vi "ktc11.vi"() -> ()   [LabVIEW 2018]
panel:
  out "RAW":dbl
  in  "stop":bool
  out "TANK":dbl(slide) scale=0.0..25.0
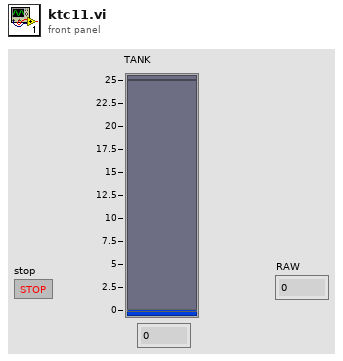
[diagram p1: front panel]
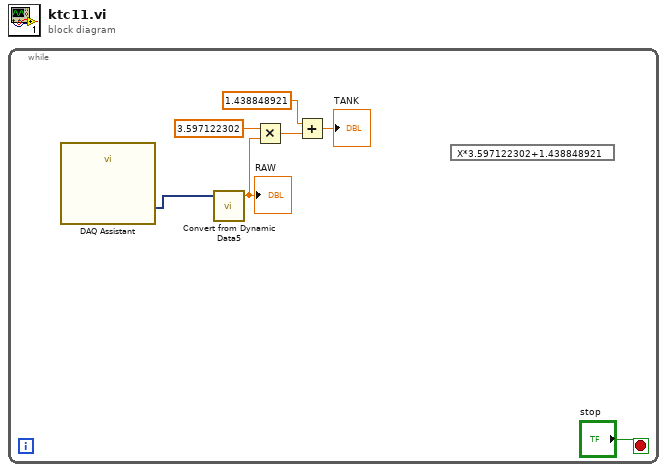
[diagram p0: block diagram]
diagram:
  n1 = while {
    stop <- "stop" stop-if-true
    n2 = call "DAQ Assistant"() -> ("data"=w6:dynamicdata)  [unwired: 17 in, 2 out]
    n3 = call "Convert from Dynamic Data5"("Dynamic Data Type"=w6) -> ("Scalar"=w5:dbl)  [unwired: 3 in]
    "RAW" <- w5
    n4 = Multiply(x=3.597122302, y=w5) -> (x*y=w3:dbl)
    n5 = Add(x=1.438848921, y=w3) -> (x+y=→"TANK":dbl)
    n6 = expression code="X*3.597122302+1.438848921"() -> ()  [unwired: 1 in, 1 out]
  }
